vi "GetValue.vi"(8 "error in":errorcluster, 11 "Int in":refnum<class "Int.lvclass">) -> (0 "error out":errorcluster, 2 "Value":i32, 3 "Int out":refnum<class "Int.lvclass">)   [LabVIEW 2021, in "ProligentXMLGenerator.lvlib" / "Int.lvclass"]
uses:
  Int.lvclass
  Int.lvclass/Int.ctl
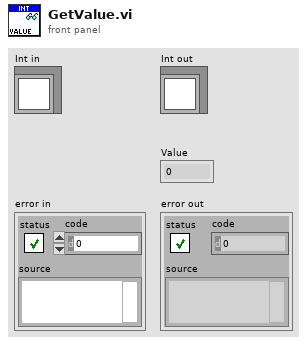
[diagram p1: front panel]
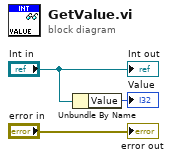
[diagram p0: block diagram]
diagram:
  n1 = Unbundle By Name("Int in") -> ("Value"=→"Value":i32)
  "error out" <- "error in"
  "Int out" <- "Int in"
